vi "Inverse_Kinematics_to_Deg_mm.vi"(3 "pz":dbl, 4 "py":dbl, 5 "px":dbl) -> (0 "L3 [mm]":dbl, 1 "L2 [deg]":dbl, 2 "L1 [deg]":dbl)   [LabVIEW 2016]
doc: "This VI converts the desired tool tip position (px,py,pz) [mm] into joint motions of theta 1, theta 2, and theta 3 [counts]."
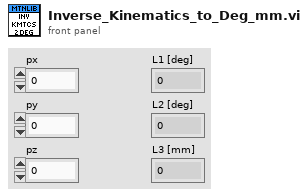
[diagram p1: front panel]
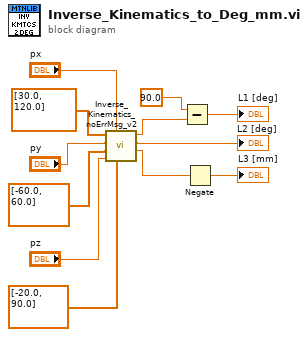
[diagram p0: block diagram]
diagram:
  n1 = call "Inverse_Kinematics_noErrMsg_v2.vi"("B3"=dbl[] [-20.0, 90.0], "px"="px", "pz"="pz", "B2"=dbl[] [-60.0, 60.0], "py"="py", "B1"=dbl[] [30.0, 120.0]) -> ("theta 3"=w5:dbl, "theta 2"=→"L2 [deg]":dbl, "theta 1"=w4:dbl)  [unwired: 1 in]
  n2 = Subtract(x=90.0, y=w4) -> (x-y=→"L1 [deg]":dbl)
  n3 = Negate(x=w5) -> (-x=→"L3 [mm]":dbl)
